vi "REQ full lifecycle v0.vi"(6 "command":T1, 7 "Julia ZMQ server file name":string="ZMQ-testserver2.jl", 8 "error in":errorcluster, 10 "data to send":string="hello", 11 "endpoint":string="tcp://127.0.0.1:5555") -> (0 "error out":errorcluster, 2 "server response":string)   [LabVIEW 2018]
uses:
  Commands.ctl
  Server or client state.ctl
  <vilib>/addons/zeromq/zmq_socket.lvclass
  <vilib>/addons/zeromq/zmq_context.lvclass
  <vilib>/Utility/error.llb/Error Cluster From Error Code.vi
  <vilib>/ErrorRing/Error Ring.xnode
  LV-Julia_ZMQ-Roundtrip_lib.lvlib
panel:
  out "cmd return code":i32
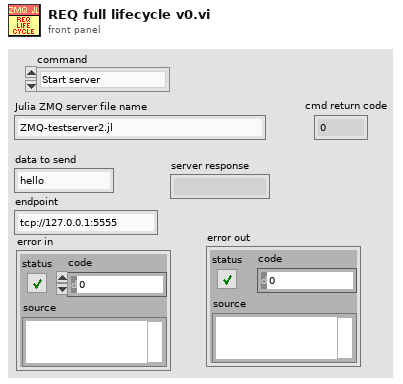
[diagram p1: front panel]
types:
  T1 = typedef "LV-Julia_ZMQ-Roundtrip_lib.lvlib/Commands.ctl" = enum16{"Start server", "Send request ", "Stop server", "Force clean-up"}
  T2 = typedef "LV-Julia_ZMQ-Roundtrip_lib.lvlib/Server or client state.ctl" = enum16{"stopped", "running", "unknown"}
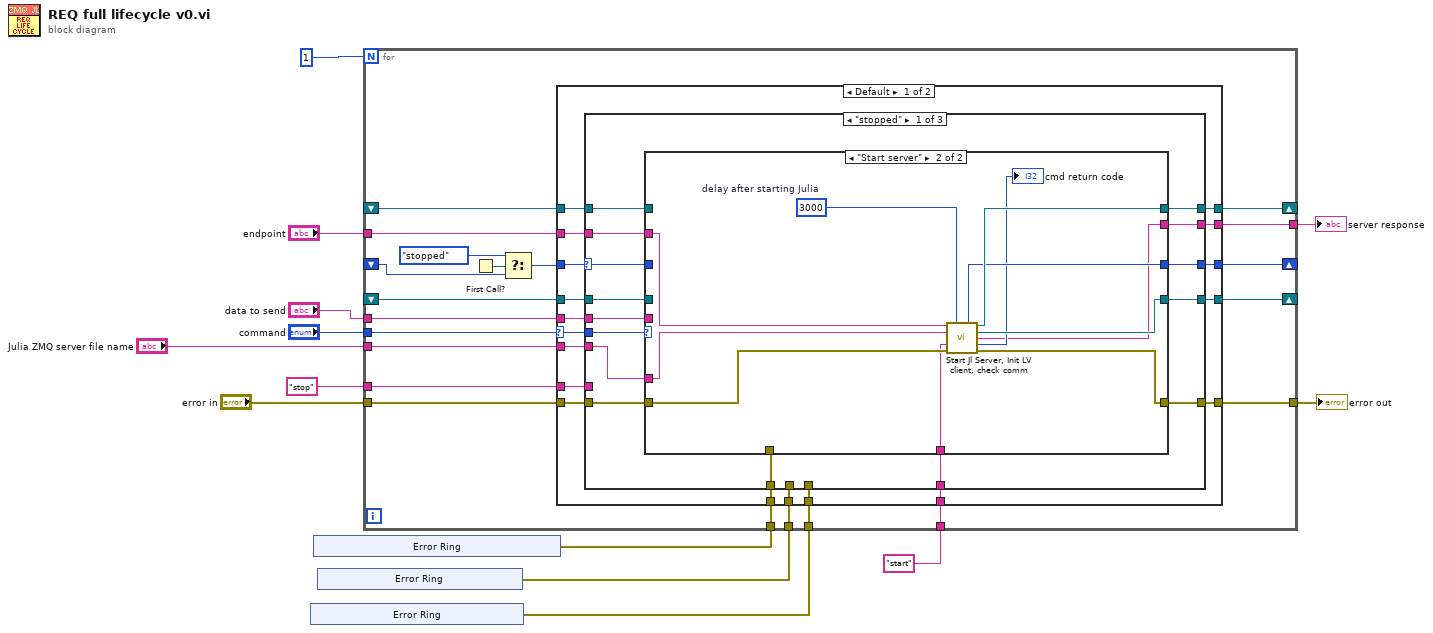
[diagram p0: block diagram]
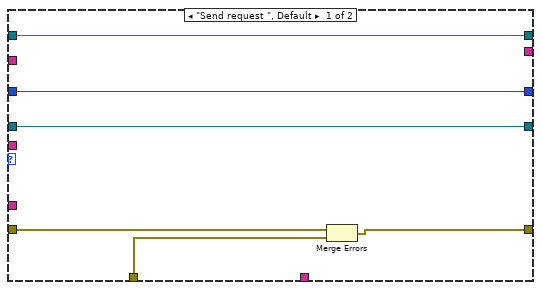
[diagram p2: hidden frame]
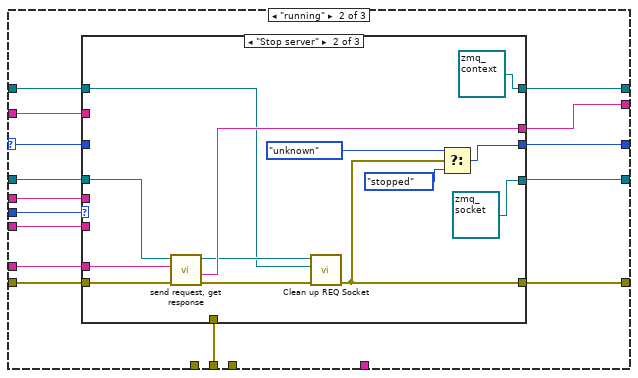
[diagram p3: hidden frame]
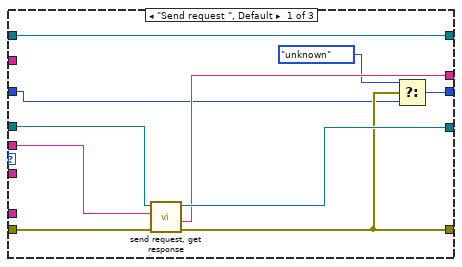
[diagram p4: hidden frame]
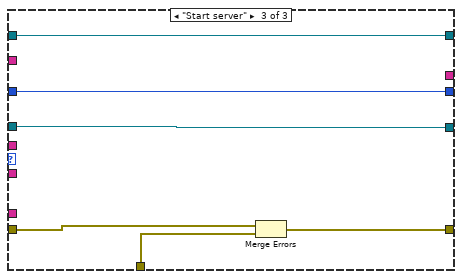
[diagram p5: hidden frame]
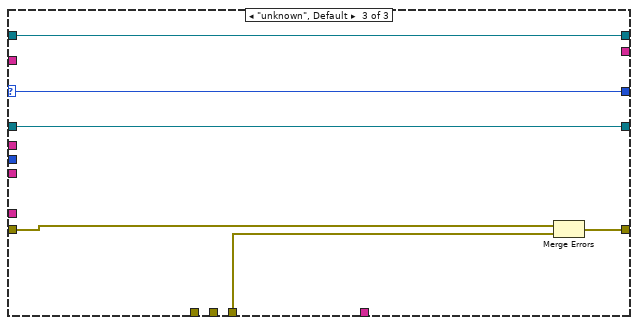
[diagram p6: hidden frame]
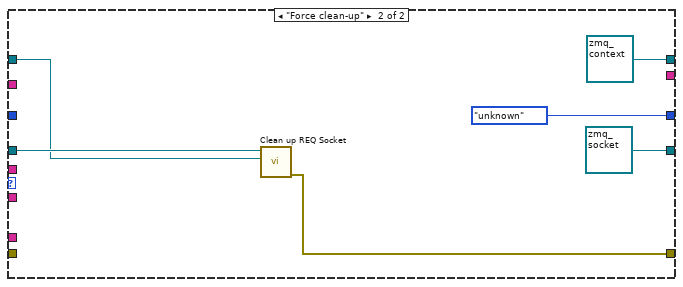
[diagram p7: hidden frame]
diagram:
  n1 = xnode "Error Ring"() -> ("error out"=w3:errorcluster)
  n2 = xnode "Error Ring"() -> ("error out"=w2:errorcluster)
  n3 = xnode "Error Ring"() -> ("error out"=w4:errorcluster)
  n4 = for {
    N: 1 -> [_]
    tunnel: [w34] -> w12
    tunnel: [w33] -> w11
    shift-right: [w32] -> _
    shift-left: _ -> [w25]
    tunnel: "endpoint" -> [w31]
    tunnel: "data to send" -> [w30]
    shift-right: [w29] -> _
    shift-left: _ -> [w24]
    tunnel: "error in" -> [w28]
    shift-right: [w26] -> _
    shift-left: _ -> [w27]
    tunnel: "command" -> [w20]
    tunnel: "Julia ZMQ server file name" -> [w19]
    tunnel: "stop" ("request") -> [w18]
    tunnel: w4 -> [w17]
    tunnel: w3 -> [w16]
    tunnel: w2 -> [w15]
    tunnel: "start" ("request") -> [w14]
    n5 = First Call?() -> (First Call?: T/F=w21:bool)
    n6 = Select(t=Server_or_client_state."stopped" ("Server state"), s=w21, f=w27) -> (s? t:f=w23:T2)
    n7 = case shown="Default" w20 {
      selector: w20 -> [w41 _]
      tunnel: [w52 w136] -> w34
      tunnel: [w51 _] -> w33
      tunnel: [w50 refnum<class "zmq_context.lvclass"> refnum ("zmq_context out")] -> w32
      tunnel: w31 -> [w49 _]
      tunnel: w30 -> [w48 _]
      tunnel: [w47 refnum<class "zmq_socket.lvclass"> refnum ("zmq_socket out")] -> w29
      tunnel: w28 -> [w46 _]
      tunnel: [w45 Server_or_client_state."unknown" ("Server state")] -> w26
      tunnel: w25 -> [w44 w137]
      tunnel: w24 -> [w43 w138]
      tunnel: w23 -> [w42 _]
      tunnel: w19 -> [w40 _]
      tunnel: w18 -> [w39 _]
      tunnel: w17 -> [w38 _]
      tunnel: w16 -> [w37 _]
      tunnel: w15 -> [w36 _]
      tunnel: w14 -> [w35 _]
      frame Default {
        n8 = case shown="\"stopped\"" w42 {
          selector: w42 -> [w54 w87 w134]
          tunnel: [w67 w99 w130] -> w52
          tunnel: [w66 w98 _] -> w51
          tunnel: [w65 w97 w133] -> w50
          tunnel: w49 -> [w64 w96 _]
          tunnel: w48 -> [w63 w95 _]
          tunnel: [w62 w94 w132] -> w47
          tunnel: w46 -> [w61 w93 w131]
          tunnel: [w59 w91 w134] -> w45
          tunnel: w44 -> [w56 w88 w133]
          tunnel: w43 -> [w57 w89 w132]
          tunnel: w41 -> [w60 w92 _]
          tunnel: w40 -> [w58 w90 _]
          tunnel: w39 -> [_ w86 _]
          tunnel: w38 -> [_ w85 _]
          tunnel: w37 -> [_ _ w129]
          tunnel: w36 -> [w55 _ _]
          tunnel: w35 -> [w53 _ _]
          frame "stopped" {
            n9 = case shown="\"Start server\"" w60 {
              tunnel: [w72 w81] -> w67
              tunnel: [_ w74] -> w66
              tunnel: [w70 w84] -> w65
              tunnel: w64 -> [_ w83]
              tunnel: w63 -> [_ _]
              tunnel: [w71 w82] -> w62
              tunnel: w61 -> [w73 w79]
              tunnel: [w68 w80] -> w59
              tunnel: w58 -> [_ w78]
              tunnel: w57 -> [w71 _]
              tunnel: w56 -> [w70 _]
              tunnel: w55 -> [w69 _]
              tunnel: w54 -> [w68 _]
              tunnel: w53 -> [_ w75]
              frame "Send request ", Default {
                n10 = Merge Errors(w73, w69) -> (w72:errorcluster)
              }
              frame "Start server" {
                w77 = u32 3000  # delay after starting Julia
                n11 = call "Start Jl Server, Init LV client, check comm.vi"("endpoint"=w83, "delay after starting Julia"=w77, "Julia ZMQ server file name"=w78, "request"=w75, "error in (no error)"=w79) -> ("JL server state"=w80:T2, "zmq_context out"=w84:refnum<class "zmq_context.lvclass">, "zmq_socket out"=w82:refnum<class "zmq_socket.lvclass">, "response"=w74:string, "return code"=→"cmd return code":i32, "error out"=w81:errorcluster)  [unwired: 4 in, 1 out]
              }
            }
          }
          frame "running" {
            n12 = case shown="\"Stop server\"" w92 {
              tunnel: [w102 w115 w124] -> w99
              tunnel: [w104 w120 _] -> w98
              tunnel: [w109 refnum<class "zmq_context.lvclass"> refnum ("zmq_context out") w128] -> w97
              tunnel: w96 -> [_ _ _]
              tunnel: w95 -> [w105 _ _]
              tunnel: [w107 refnum<class "zmq_socket.lvclass"> refnum ("zmq_socket out") w127] -> w94
              tunnel: w93 -> [w108 w122 w126]
              tunnel: [w101 w118 w125] -> w91
              tunnel: w90 -> [_ _ _]
              tunnel: w89 -> [w106 w121 w127]
              tunnel: w88 -> [w109 w112 w128]
              tunnel: w87 -> [w100 _ w125]
              tunnel: w86 -> [_ w117 _]
              tunnel: w85 -> [_ _ w123]
              frame "Send request ", Default {
                n13 = call "send request, get response.vi"("error in (no error)"=w108, "request"=w105, "zmq_socket in"=w106) -> ("error out"=w102:errorcluster, "response"=w104:string, "zmq_socket out"=w107:refnum<class "zmq_socket.lvclass">)  [unwired: 4 in, 2 out]
                n14 = Select(t=Server_or_client_state."unknown" ("Server state"), s=w102, f=w100) -> (s? t:f=w101:T2)
              }
              frame "Stop server" {
                n15 = call "send request, get response.vi"("error in (no error)"=w122, "request"=w117, "zmq_socket in"=w121) -> ("error out"=w116:errorcluster, "response"=w120:string, "zmq_socket out"=w113:refnum<class "zmq_socket.lvclass">)  [unwired: 4 in, 2 out]
                n16 = call "Clean up REQ Socket.vi"("error in (no error)"=w116, "zmq_context in"=w112, "zmq_socket in"=w113) -> ("error out"=w115:errorcluster)  [unwired: 8 in]
                n17 = Select(t=Server_or_client_state."unknown" ("Server state"), s=w115, f=Server_or_client_state."stopped") -> (s? t:f=w118:T2)
              }
              frame "Start server" {
                n18 = Merge Errors(w126, w123) -> (w124:errorcluster)
              }
            }
          }
          frame "unknown", Default {
            n19 = Merge Errors(w131, w129) -> (w130:errorcluster)
          }
        }
      }
      frame "Force clean-up" {
        n20 = call "Clean up REQ Socket.vi"("zmq_context in"=w137, "zmq_socket in"=w138) -> ("error out"=w136:errorcluster)  [unwired: 9 in]
      }
    }
  }
  "error out" <- w12
  "server response" <- w11
